vi "PS Control.vi"(11 "Message Enqueuer":refnum<class "Message Enqueuer.lvclass">) -> ()   [LabVIEW 2024, in "PS Control Persistence.lvlib"]
uses:
  PS Control Persistence.lvlib
  <vilib>/ActorFramework/Message Enqueuer/Message Enqueuer.lvclass
  <vilib>/ActorFramework/Message Enqueuer/Message Enqueuer.lvclass/Message Enqueuer.ctl
  PS Control Actor Messages/Write Staff mode Msg/Write Staff mode Msg.lvclass/Write Staff mode Msg.ctl
  PS Control Actor Messages/Choose configuration mode Msg/Choose configuration mode Msg.lvclass/Choose configuration mode Msg.ctl
  PS Control Actor Messages/Change VISA address Msg/Change VISA address Msg.lvclass/Change VISA address Msg.ctl
  PS Control Actor Messages/Setpoint Msg/Setpoint Msg.lvclass/Setpoint Msg.ctl
  <vilib>/ActorFramework/Message Enqueuer/Enqueue.vi
  PS Control Actor Messages/RampToSetpoint Msg/RampToSetpoint Msg.lvclass
  C:/Program Files/National Instruments/LabVIEW 2024/vi.lib/ActorFramework/Message/Message.lvclass
  PS Control Actor Messages/Write Staff mode Msg/Write Staff mode Msg.lvclass
  PS Control Actor Messages/Choose configuration mode Msg/Choose configuration mode Msg.lvclass
  PS Control Actor Messages/Hold Msg/Hold Msg.lvclass
  PS Control Actor Messages/Change VISA address Msg/Change VISA address Msg.lvclass
  PS Control Persistence Actor Messages/Make persistent Msg/Make persistent Msg.lvclass
  PS Control Persistence Actor Messages/Make unpersistent Msg/Make unpersistent Msg.lvclass
  PS Control Actor Messages/RampToZero Msg/RampToZero Msg.lvclass
  PS Control Actor Messages/Setpoint Msg/Setpoint Msg.lvclass
  <vilib>/ActorFramework/Stop Msg/Stop Msg.lvclass
  <vilib>/ActorFramework/Message Priority Queue/Priority Enqueue.vi
panel:
  out "Persistence Status":string
  out "Persistent":bool
  in  "Return from persistence":bool
  in  "Make Persistent":bool
  out "Switch Heater\nError":bool
  out "Switch heater \nconfirmed":bool
  out "Switch Heater":bool
  out "Status":string
  in  "Operating mode":u16(ring) items=["Normal"]
  in  "Staff mode":bool
  out "error out":errorcluster
  in  "VISA address":refnum<visa-resource-name>="GPIB0::22::INSTR"
  in  "stop":bool
  in  "Ramp to Zero":bool
  in  "Hold":bool
  in  "Ramp to Setpoint":bool
  in  "Slew Rate [T/min]":dbl min=0.0 max=5.0 step=0.1 format="%_5f"
  in  "Setpoint [T]":dbl format="%.3f"
  out "Magnet\nVoltage":dbl format="%.2f"
  out "Field [T]":dbl format="%.4f"
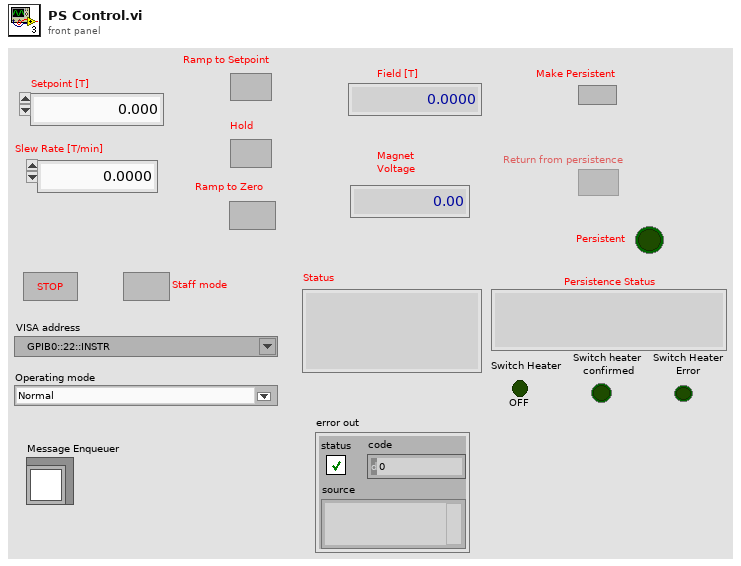
[diagram p1: front panel]
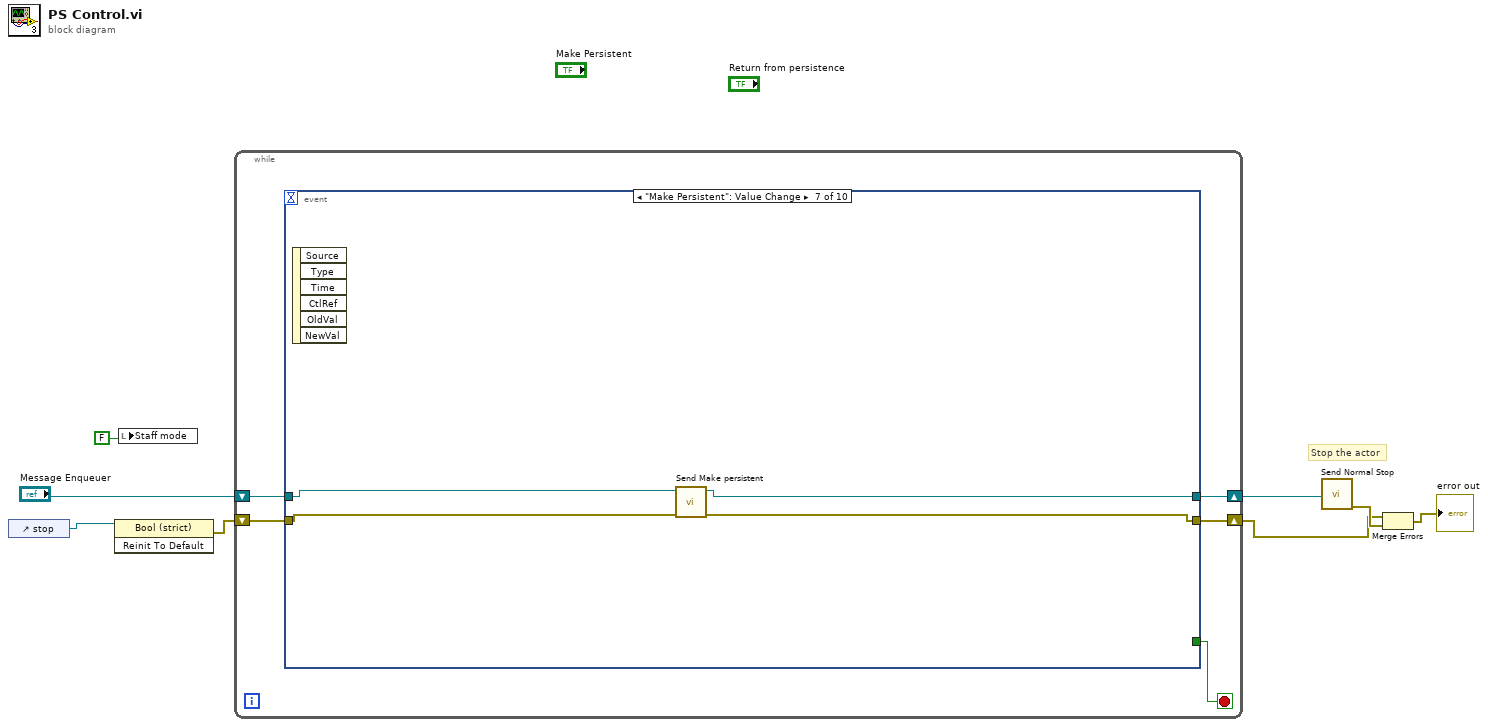
[diagram p0: block diagram]
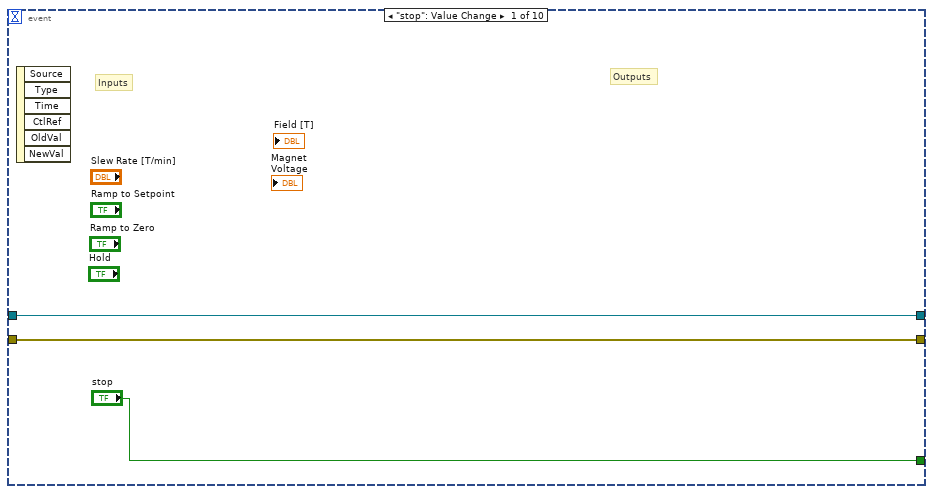
[diagram p2: hidden frame]
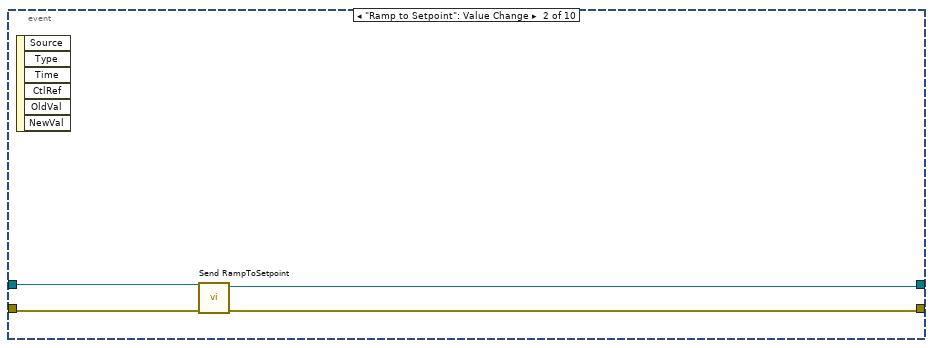
[diagram p3: hidden frame]
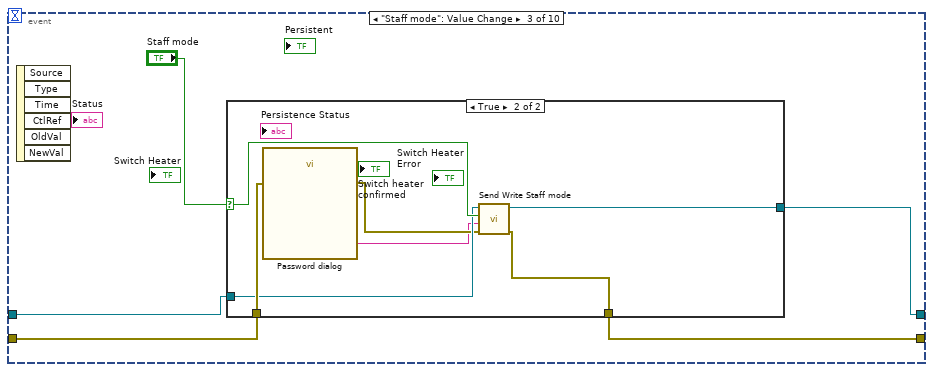
[diagram p4: hidden frame]
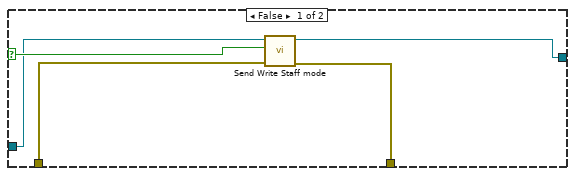
[diagram p5: hidden frame]
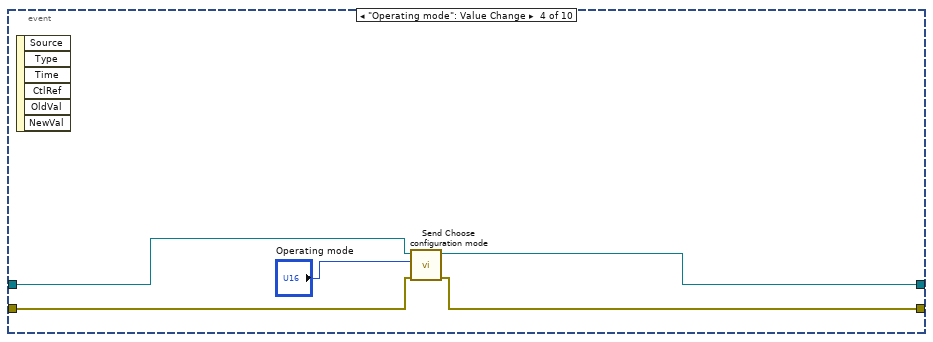
[diagram p6: hidden frame]
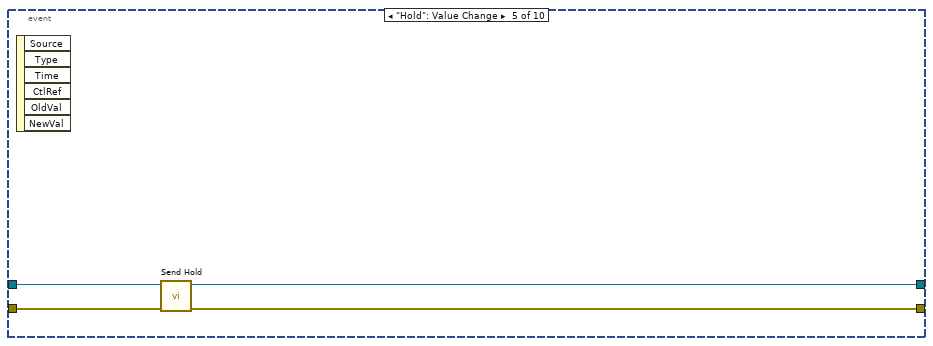
[diagram p7: hidden frame]
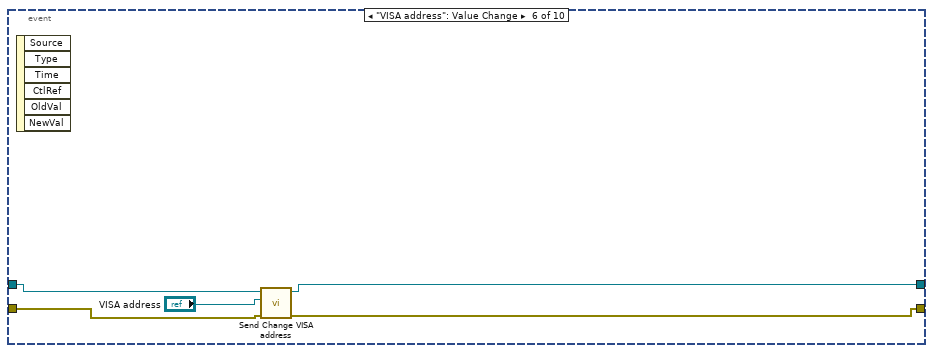
[diagram p8: hidden frame]
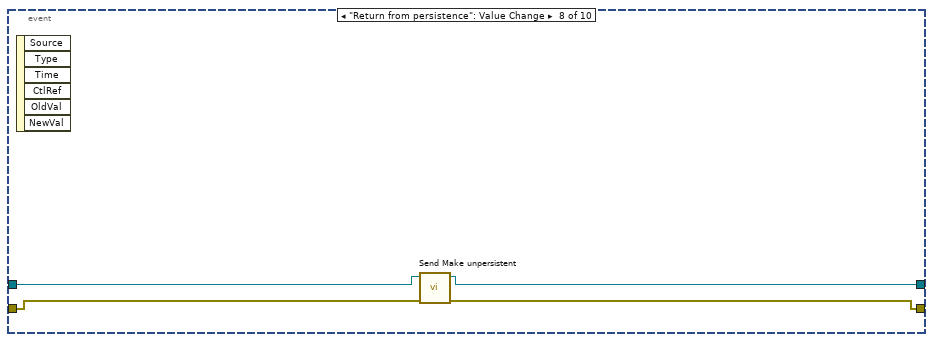
[diagram p9: hidden frame]
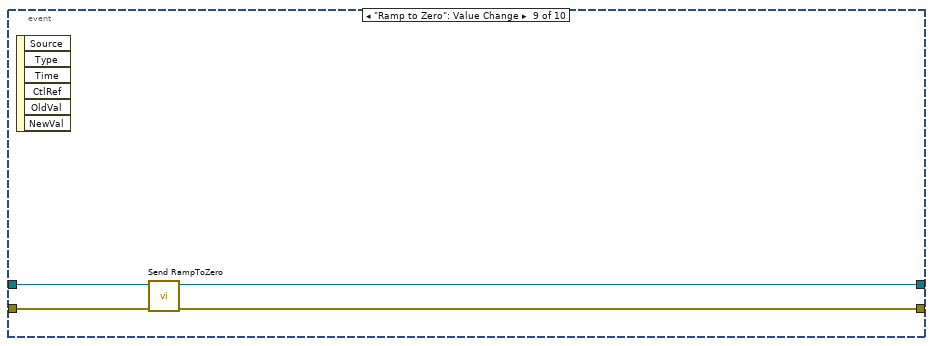
[diagram p10: hidden frame]
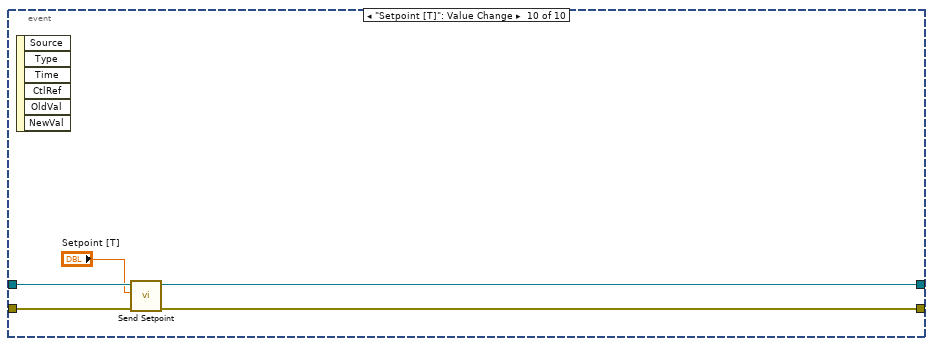
[diagram p11: hidden frame]
diagram:
  # "Stop the actor"
  n1 = control-ref of="stop"() -> (w8:refnum<vi>)
  n2 = invoke class="Bool (strict)" method="Reinit To Default"(reference=w8) -> (error out=w2:errorcluster)  [unwired: 2 in, 2 out]
  n3 = local write "Staff mode"(FALSE ("Staff mode")) -> ()
  n4 = while {
    shift-right: [w10] -> w7
    shift-left: "Message Enqueuer" -> [w12]
    shift-right: [w9] -> w3
    shift-left: w2 -> [w13]
    stop <- w11 stop-if-true
    n5 = event shown="[6] \"Make Persistent\": Value Change" {
      selector: _ -> [_ _ _ _ _ _ _ _ _ _]
      dyn-events: _ -> [_ _ _ _ _ _ _ _ _ _]
      timeout: _ -> [_ _ _ _ _ _ _ _ _ _]
      tunnel: ["stop" _ _ _ _ _ _ _ _ _] -> w11
      tunnel: w13 -> [w14 w19 w23 w40 w45 w49 w54 w56 w62 w67]
      tunnel: [w15 w17 w21 w38 w44 w48 w53 w58 w60 w65] -> w10
      tunnel: w12 -> [w15 w20 w22 w41 w46 w50 w55 w57 w63 w68]
      tunnel: [w14 w18 w24 w39 w43 w47 w52 w59 w61 w64] -> w9
      event "stop": Value Change {
        # "Outputs"
        # "Inputs"
        n6 = event-data() -> ()  [unwired: 1 in, 6 out]
      }
      event "Ramp to Setpoint": Value Change {
        n7 = event-data() -> ()  [unwired: 1 in, 6 out]
        n8 = call "Send RampToSetpoint.vi"("error in (no error)"=w19, "Message Enqueuer"=w20) -> ("error out"=w18:errorcluster, "Message Enqueuer out"=w17:refnum<class "Message Enqueuer.lvclass">)  [unwired: 8 in]
      }
      event "Staff mode": Value Change {
        n9 = event-data() -> ()  [unwired: 1 in, 6 out]
        n10 = case shown="True" "Staff mode" {
          selector: "Staff mode" -> [w29 w36]
          tunnel: [w27 w33] -> w24
          tunnel: w23 -> [w30 w37]
          tunnel: w22 -> [w28 w35]
          tunnel: [w26 w34] -> w21
          frame False {
            n11 = call "Send Write Staff mode.vi"("error in (no error)"=w30, "Staff mode"=w29, "Message Enqueuer"=w28) -> ("error out"=w27:errorcluster, "Message Enqueuer out"=w26:refnum<class "Message Enqueuer.lvclass">)  [unwired: 7 in]
          }
          frame True {
            n12 = call "Password dialog.vi"("error in (no error)"=w37) -> ("Password"=w31:string, "error out"=w32:errorcluster)  [unwired: 16 in, 1 out]
            n13 = call "Send Write Staff mode.vi"("error in (no error)"=w32, "Password"=w31, "Staff mode"=w36, "Message Enqueuer"=w35) -> ("error out"=w33:errorcluster, "Message Enqueuer out"=w34:refnum<class "Message Enqueuer.lvclass">)  [unwired: 6 in]
          }
        }
      }
      event "Operating mode": Value Change {
        n14 = event-data() -> ()  [unwired: 1 in, 6 out]
        n15 = call "Send Choose configuration mode.vi"("error in (no error)"=w40, "Choose configuration mode"="Operating mode", "Message Enqueuer"=w41) -> ("error out"=w39:errorcluster, "Message Enqueuer out"=w38:refnum<class "Message Enqueuer.lvclass">)  [unwired: 7 in]
      }
      event "Hold": Value Change {
        n16 = event-data() -> ()  [unwired: 1 in, 6 out]
        n17 = call "Send Hold.vi"("error in (no error)"=w45, "Message Enqueuer"=w46) -> ("error out"=w43:errorcluster, "Message Enqueuer out"=w44:refnum<class "Message Enqueuer.lvclass">)  [unwired: 8 in]
      }
      event "VISA address": Value Change {
        n18 = event-data() -> ()  [unwired: 1 in, 6 out]
        n19 = call "Send Change VISA address.vi"("error in (no error)"=w49, "VISA address"="VISA address", "Message Enqueuer"=w50) -> ("error out"=w47:errorcluster, "Message Enqueuer out"=w48:refnum<class "Message Enqueuer.lvclass">)  [unwired: 7 in]
      }
      event "Make Persistent": Value Change {
        n20 = event-data() -> ()  [unwired: 1 in, 6 out]
        n21 = call "Send Make persistent.vi"("error in (no error)"=w54, "Message Enqueuer"=w55) -> ("error out"=w52:errorcluster, "Message Enqueuer out"=w53:refnum<class "Message Enqueuer.lvclass">)  [unwired: 8 in]
      }
      event "Return from persistence": Value Change {
        n22 = event-data() -> ()  [unwired: 1 in, 6 out]
        n23 = call "Send Make unpersistent.vi"("error in (no error)"=w56, "Message Enqueuer"=w57) -> ("error out"=w59:errorcluster, "Message Enqueuer out"=w58:refnum<class "Message Enqueuer.lvclass">)  [unwired: 8 in]
      }
      event "Ramp to Zero": Value Change {
        n24 = event-data() -> ()  [unwired: 1 in, 6 out]
        n25 = call "Send RampToZero.vi"("error in (no error)"=w62, "Message Enqueuer"=w63) -> ("error out"=w61:errorcluster, "Message Enqueuer out"=w60:refnum<class "Message Enqueuer.lvclass">)  [unwired: 8 in]
      }
      event "Setpoint [T]": Value Change {
        n26 = event-data() -> ()  [unwired: 1 in, 6 out]
        n27 = call "Send Setpoint.vi"("error in (no error)"=w67, "Setpoint [T]"="Setpoint [T]", "Message Enqueuer"=w68) -> ("error out"=w64:errorcluster, "Message Enqueuer out"=w65:refnum<class "Message Enqueuer.lvclass">)  [unwired: 7 in]
      }
    }
  }
  n28 = call <vilib>:"Send Normal Stop.vi"("Message Enqueuer"=w7) -> ("error out"=w4:errorcluster)  [unwired: 10 in]
  n29 = Merge Errors(w3, w4) -> (→"error out":errorcluster)
